vi "DEMO.vi"() -> ()   [LabVIEW 2013]
uses:
  Caffee.lvclass/Coffee.lvclass
  Tea.lvclass/Tea.lvclass
  CaffeineBeverage.lvclass/CaffeineBeverage.lvclass
panel:
  out "茶的泡法":string
  out "咖啡的泡法":string
  # "樣板方法模式"
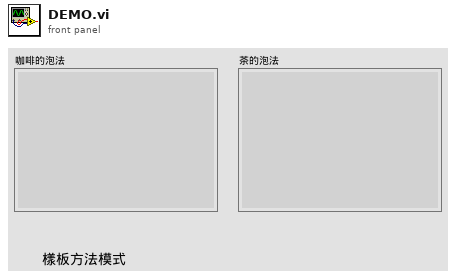
[diagram p1: front panel]
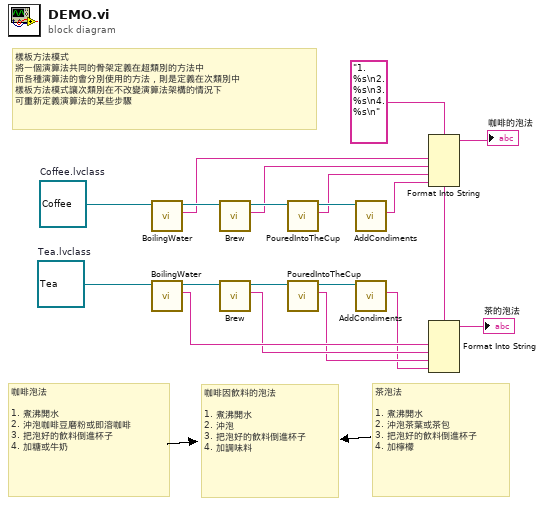
[diagram p0: block diagram]
diagram:
  w7 = "1. %s\n2. %s\n3. %s\n4. %s\n" ("format string")
  w12 = refnum<class "Tea.lvclass"> refnum  # Tea.lvclass
  w16 = refnum<class "Coffee.lvclass"> refnum  # Coffee.lvclass
  # "咖啡因飲料的泡法\n\n1. 煮沸開水\n2. 沖泡\n3. 把泡好的飲料倒進杯子\n4. 加調味料"
  # "茶泡法\n\n1. 煮沸開水\n2. 沖泡茶葉或茶包\n3. 把泡好的飲料倒進杯子\n4. 加檸檬"
  # "咖啡泡法\n\n1. 煮沸開水\n2. 沖泡咖啡豆磨粉或即溶咖啡\n3. 把泡好的飲料倒進杯子\n4. 加糖或牛奶"
  # "樣板方法模式\n將一個演算法共同的骨架定義在超類別的方法中\n而各種演算法的會分別使用的方法，則是定義在次類別中\n樣板方法模式讓次類別在不改變演算法架構的情況下\n可重新定義演算法的某些步驟"
  n1 = call "BoilingWater.vi"("CaffeineBeverage in"=w16) -> ("ProcessMessage"=w11:string, "CaffeineBeverage out"=w19:refnum<class "Coffee.lvclass">)  [unwired: 8 in, 1 out]
  n2 = call "BoilingWater.vi"("CaffeineBeverage in"=w12) -> ("ProcessMessage"=w6:string, "CaffeineBeverage out"=w13:refnum<class "Tea.lvclass">)  [unwired: 8 in, 1 out]
  n3 = call-dynamic "Brew.vi"("Coffee in"=w19) -> ("ProcessMessage"=w10:string, "Coffee out"=w18:refnum<class "Coffee.lvclass">)  [unwired: 8 in, 1 out]
  n4 = call-dynamic "Brew.vi"("Tea in"=w13) -> ("ProcessMessage"=w5:string, "Tea out"=w14:refnum<class "Tea.lvclass">)  [unwired: 8 in, 1 out]
  n5 = call "PouredIntoTheCup.vi"("CaffeineBeverage in"=w18) -> ("ProcessMessage"=w9:string, "CaffeineBeverage out"=w17:refnum<class "Coffee.lvclass">)  [unwired: 8 in, 1 out]
  n6 = call "PouredIntoTheCup.vi"("CaffeineBeverage in"=w14) -> ("ProcessMessage"=w4:string, "CaffeineBeverage out"=w15:refnum<class "Tea.lvclass">)  [unwired: 8 in, 1 out]
  n7 = call-dynamic "AddCondiments.vi"("Coffee in"=w17) -> ("ProcessMessage"=w8:string)  [unwired: 8 in, 2 out]
  n8 = call-dynamic "AddCondiments.vi"("Tea in"=w15) -> ("ProcessMessage"=w3:string)  [unwired: 8 in, 2 out]
  n9 = Format Into String(format string=w7, w11, w10, w9, w8) -> (resulting string=→"咖啡的泡法":string)  [unwired: 2 in, 1 out]
  n10 = Format Into String(format string=w7, w6, w5, w4, w3) -> (resulting string=→"茶的泡法":string)  [unwired: 2 in, 1 out]
